vi "Find Ball.vi"(0 "Search Mode":u16) -> ()   [LabVIEW 2013]
uses:
  Robot Global Data.vi
panel:
  in  "Spin Duration (ms)":u16=1000
  in  "Spin Speed":dbl=1.0
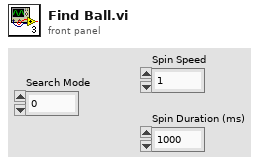
[diagram p1: front panel]
types:
  T1 = enum16{"Hold", "Pick Up", "Catch", "Aim", "Shoot", "Joystick"}
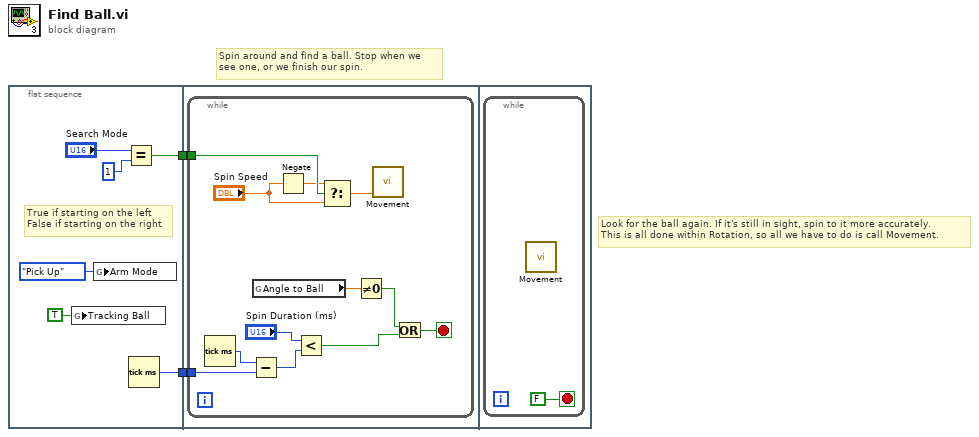
[diagram p0: block diagram]
diagram:
  # "Look for the ball again. If it's still in sight, spin to it more accurately.\nThis is all done within Rotation, so all we have to do is call Movement."
  # "Spin around and find a ball. Stop when we see one, or we finish our spin."
  n1 = flat-sequence {
    tunnel: [w5] -> w2
    tunnel: [w8] -> w1
    tunnel: w2 -> [w10]
    tunnel: w1 -> [w9]
    frame #0 {
      # "True if starting on the left\nFalse if starting on the right"
      n2 = global write "Robot Global Data.vi" "Tracking Ball"(TRUE ("Tracking Ball")) -> ()
      n3 = global write "Robot Global Data.vi" "Arm Mode"(T1."Pick Up" ("Arm Mode")) -> ()
      n4 = Equal?(x="Search Mode", y=u16 1) -> (x = y?=w5:bool)
      n5 = Tick Count (ms)() -> (millisecond timer value=w8:u32)
    }
    frame #1 {
      n6 = while {
        tunnel: w10 -> [w22]
        tunnel: w9 -> [w19]
        stop <- w15 stop-if-true
        n7 = Tick Count (ms)() -> (millisecond timer value=w20:u32)
        n8 = Subtract(x=w20, y=w19) -> (x-y=w17:u32)
        n9 = global read "Robot Global Data.vi" "Angle to Ball"() -> (w14:dbl)
        n10 = Negate(x="Spin Speed") -> (-x=w11:dbl)
        n11 = Less?(x="Spin Duration (ms)", y=w17) -> (x < y?=w16:bool)
        n12 = Select(t=w11, s=w22, f="Spin Speed") -> (s? t:f=w21:dbl)
        n13 = Not Equal To 0?(x=w14) -> (x != 0?=w13:bool)
        n14 = call "Movement.vi"("Rotational Speed"=w21) -> ()  [unwired: 2 in]
        n15 = Or(x=w13, y=w16) -> (x .or. y?=w15:bool)
      }
    }
    frame #2 {
      n16 = while {
        stop <- FALSE stop-if-true
        n17 = call "Movement.vi"() -> ()  [unwired: 3 in]
      }
    }
  }
